vi "open vi.vi"(10 "error in":errorcluster, 11 "vi path":path) -> (2 "error out":errorcluster)   [LabVIEW 2022 SP3]
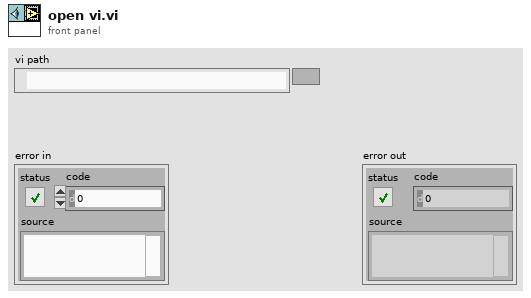
[diagram p1: front panel]
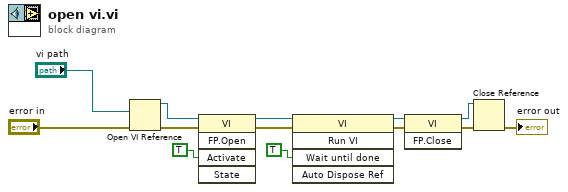
[diagram p0: block diagram]
diagram:
  n1 = Open VI Reference(vi path="vi path", error in (no error)="error in") -> (vi reference=w12:refnum<vi>, error out=w11:errorcluster)  [unwired: 4 in]
  n2 = invoke class="VI" method="FP.Open"(reference=w12, error in=w11, "Activate"=TRUE ("Activate?")) -> (reference out=w9:refnum<vi>, error out=w8:errorcluster)  [unwired: 2 in, 3 out]
  n3 = invoke class="VI" method="Run VI"(reference=w9, error in=w8, "Wait until done"=TRUE ("Wait Until Done")) -> (reference out=w6:refnum<vi>, error out=w5:errorcluster)  [unwired: 2 in, 3 out]
  n4 = invoke class="VI" method="FP.Close"(reference=w6, error in=w5) -> (reference out=w4:refnum<vi>, error out=w3:errorcluster)  [unwired: 1 in, 1 out]
  n5 = Close Reference(reference=w4, error in (no error)=w3) -> (error out=→"error out":errorcluster)
